vi "CTR_DAQSensorConfigs.vi"(8 "error in":errorcluster, 10 "Sensors in":T1(array[cluster]), 11 "node in":refnum<k20>) -> (0 "error out":errorcluster={"status"=TRUE, "code"=-2633, "source"="Property Node (arg 1) in NI_XML.lvlib:Get Node Text Content.vi->CTR_ControlNodeConfigs.vi->CTR_ReadXML_Config.vi->CTRnode.vi"}, 2 "Sensors out":T1(array[cluster]), 3 "node out":refnum<k20>)   [LabVIEW 2024]
uses:
  <vilib>/xml/Close Reference(Node).vi
  <vilib>/xml/NI_XML.lvlib
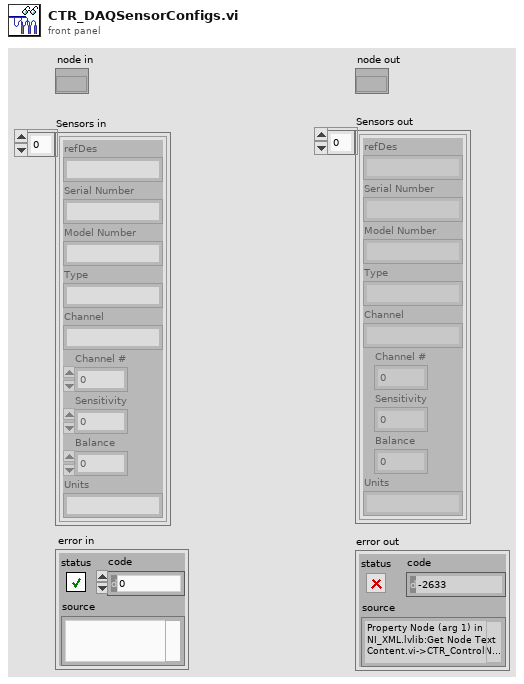
[diagram p1: front panel]
types:
  T1 = cluster{"refDes":string, "Serial Number":string, "Model Number":string, "Type":string, "Channel":string, "Channel #":i32, "Sensitivity":dbl, "Balance":dbl, "Units":string}[]
  T2 = cluster{"refDes":string, "Serial Number":string, "Model Number":string, "Type":string, "Channel":string, "Channel #":i32, "Sensitivity":dbl, "Balance":dbl, "Units":string}
  T3 = cluster{"[0]":string, "[1]":string, "[2]":string, "[3]":string, "[4]":string, "[5]":string, "[6]":string, "[7]":string, "[8]":string}
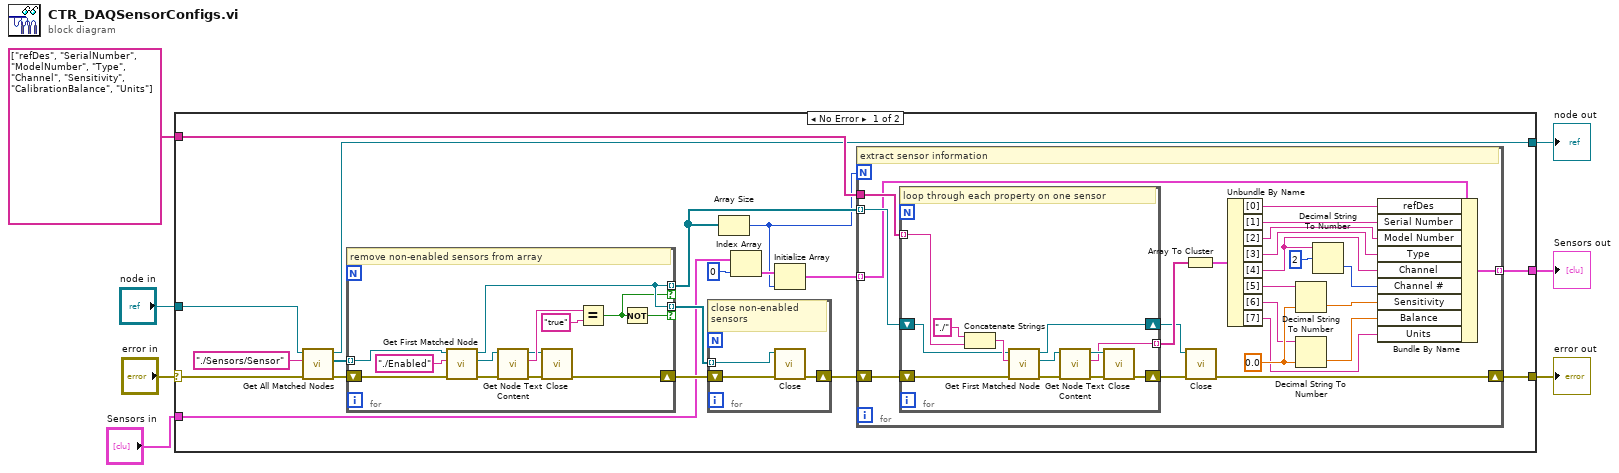
[diagram p0: block diagram]
diagram:
  n1 = case shown="No Error" "error in" {
    selector: "error in" -> [w25 w79]
    tunnel: [w24 w79] -> w6
    tunnel: "node in" -> [w22 w78]
    tunnel: string[] ["refDes", "SerialNumber", "ModelNumber", "Type", "Channel", "Sensitivity", "CalibrationBalance", "Units"] -> [w21 _]
    tunnel: [w13 w78] -> w7
    tunnel: "Sensors in" -> [w9 w77]
    tunnel: [w8 w77] -> w1
    frame No Error {
      n2 = call <vilib>:"Get All Matched Nodes.vi"("error in (no error)"=w25, "XPath expression"="./Sensors/Sensor" ("string"), "node in"=w22) -> ("error out"=w17:errorcluster, "node result array"=w14:refnum<k20>[], "node out"=w13:refnum<k20>)  [unwired: 6 in]
      n3 = for {
        shift-right: [w33] -> w19
        shift-left: w17 -> [w34]
        tunnel: [w32] -> w15 mode=indexing if=w30
        tunnel: [w32] -> w18 mode=indexing if=w31
        tunnel: w14 -> [w29] mode=indexing
        # "remove non-enabled sensors from array"
        n4 = call <vilib>:"Get First Matched Node.vi"("error in (no error)"=w34, "XPath expression"="./Enabled", "node in"=w29) -> ("error out"=w37:errorcluster, "node result"=w38:refnum<k20>, "node out"=w32:refnum<k20>)  [unwired: 6 in]
        n5 = call <vilib>:"Get Node Text Content.vi"("error in (no error)"=w37, "node in"=w38) -> ("error out"=w39:errorcluster, "node text"=w41:string, "node out"=w40:refnum<k20>)  [unwired: 7 in]
        n6 = call-poly <vilib>:"Close.vi"("error in (no error)"=w39, "node"=w40) -> ("error out"=w33:errorcluster)  [unwired: 7 in]
        n7 = Equal?(x=w41, y="true" ("x")) -> (x = y?=w30:bool)
        n8 = Not(x=w30) -> (.not. x?=w31:bool)
      }
      n9 = for {
        tunnel: w18 -> [w28] mode=indexing
        shift-right: [w26] -> w16
        shift-left: w19 -> [w27]
        # "close non-enabled sensors"
        n10 = call-poly <vilib>:"Close.vi"("error in (no error)"=w27, "node"=w28) -> ("error out"=w26:errorcluster)  [unwired: 7 in]
      }
      n11 = Array Size(array=w15) -> (size(s)=w11:i32)
      n12 = Index Array(array=w9, index=0) -> (element=w12:T2)
      n13 = Initialize Array(w12, w11) -> (w10:T1)
      n14 = for {
        N: w11 -> [_]
        shift-right: [w56] -> w24
        shift-left: w16 -> [w63]
        tunnel: w21 -> [w64]
        tunnel: w15 -> [w62] mode=indexing
        tunnel: w10 -> [w61] mode=indexing
        tunnel: [w55] -> w8 mode=indexing
        w49 = 0.0
        # "extract sensor information"
        n15 = for {
          tunnel: w64 -> [w70] mode=indexing
          shift-right: [w65] -> w57
          shift-left: w63 -> [w72]
          shift-right: [w67] -> w58
          shift-left: w62 -> [w68]
          tunnel: [w66] -> w60 mode=indexing
          # "loop through each property on one sensor"
          n16 = Concatenate Strings("./" ("string"), w70) -> (w69:string)
          n17 = call <vilib>:"Get First Matched Node.vi"("error in (no error)"=w72, "XPath expression"=w69, "node in"=w68) -> ("error out"=w76:errorcluster, "node result"=w75:refnum<k20>, "node out"=w67:refnum<k20>)  [unwired: 6 in]
          n18 = call <vilib>:"Get Node Text Content.vi"("error in (no error)"=w76, "node in"=w75) -> ("error out"=w74:errorcluster, "node text"=w66:string, "node out"=w73:refnum<k20>)  [unwired: 7 in]
          n19 = call-poly <vilib>:"Close.vi"("error in (no error)"=w74, "node"=w73) -> ("error out"=w65:errorcluster)  [unwired: 7 out]
        }
        n20 = Array To Cluster(array=w60) -> (cluster=w59:T3)
        n21 = call-poly <vilib>:"Close.vi"("error in (no error)"=w57, "node"=w58) -> ("error out"=w56:errorcluster)  [unwired: 7 out]
        n22 = Unbundle By Name(w59) -> ("[0]"=w54:string, "[1]"=w53:string, "[2]"=w52:string, "[3]"=w51:string, "[4]"=w46:string, "[5]"=w45:string, "[6]"=w44:string, "[7]"=w43:string)
        n23 = Decimal String To Number(string=w45, default (0L)=w49) -> (number=w47:dbl)  [unwired: 1 in, 1 out]
        n24 = Decimal String To Number(string=w44, default (0L)=w49) -> (number=w48:dbl)  [unwired: 1 in, 1 out]
        n25 = Decimal String To Number(string=w46, offset=2 ("default (0 I32)")) -> (number=w50:i32)  [unwired: 1 in, 1 out]
        n26 = Bundle By Name(cluster=w61, "refDes"=w54, "Serial Number"=w53, "Model Number"=w52, "Type"=w51, "Channel"=w46, "Channel #"=w50, "Sensitivity"=w47, "Balance"=w48, "Units"=w43) -> (w55:T2)
      }
    }
    frame Error {
    }
  }
  "error out" <- w6
  "node out" <- w7
  "Sensors out" <- w1
